vi "Read state.vi"(8 "error in (no error)":errorcluster, 11 "GuideAutoclearState in":refnum<class "GuideAutoclearState.lvclass">) -> (0 "error out":errorcluster, 2 "guideAutoclearStateTypes":T1, 3 "GuideAutoclearState out":refnum<class "GuideAutoclearState.lvclass">)   [LabVIEW 2014, in "TCSDataDefinitions.lvlib" / "TCSCommand.lvlib" / "GuiderCommands.lvlib" / "GuideAutoclearState.lvclass"]
uses:
  GuideAutoclearState.lvclass
  Enumerations/GuideAutoclearStateTypes.ctl
  GuideAutoclearState.lvclass/GuideAutoclearState.ctl
  TCSCommand.lvlib
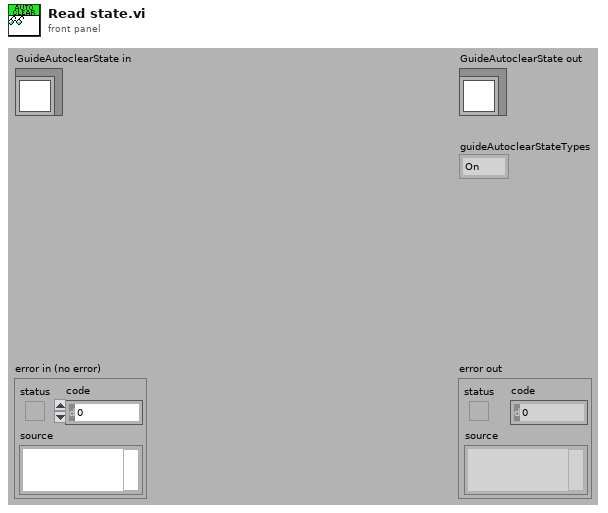
[diagram p1: front panel]
types:
  T1 = typedef "TCSDataDefinitions.lvlib/TCSCommand.lvlib/GuideAutoclearStateTypes.ctl" = enum16{"On", "Off"}
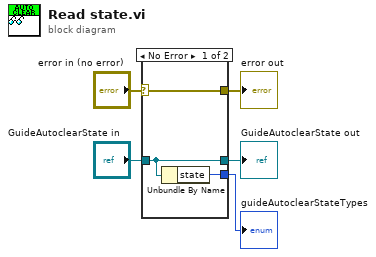
[diagram p0: block diagram]
diagram:
  n1 = case shown="No Error" "error in (no error)" {
    selector: "error in (no error)" -> [w8 w9]
    tunnel: [w8 w9] -> w4
    tunnel: [w7 w10] -> w2
    tunnel: "GuideAutoclearState in" -> [w7 w10]
    tunnel: [w6 _] -> w1
    frame No Error {
      n2 = Unbundle By Name(w7) -> ("state"=w6:T1)
    }
    frame Error {
    }
  }
  "error out" <- w4
  "GuideAutoclearState out" <- w2
  "guideAutoclearStateTypes" <- w1
